vi "Terminals - Filter Left-Top Term.vi"(11 "Terms[]":refnum<vi>[](array[refnum])) -> (3 "Terms[] out":refnum<vi>[](array[refnum]))   [LabVIEW 2020, in "CSM-Helper.lvclass"]
uses:
  CSM-Helper.lvclass
  CSM-Helper.lvclass/CSM-Helper.ctl
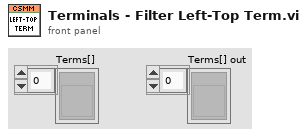
[diagram p1: front panel]
types:
  T1 = typedef "LVPositionTypeDef.ctl" = cluster{"Left":i32, "Top":i32}
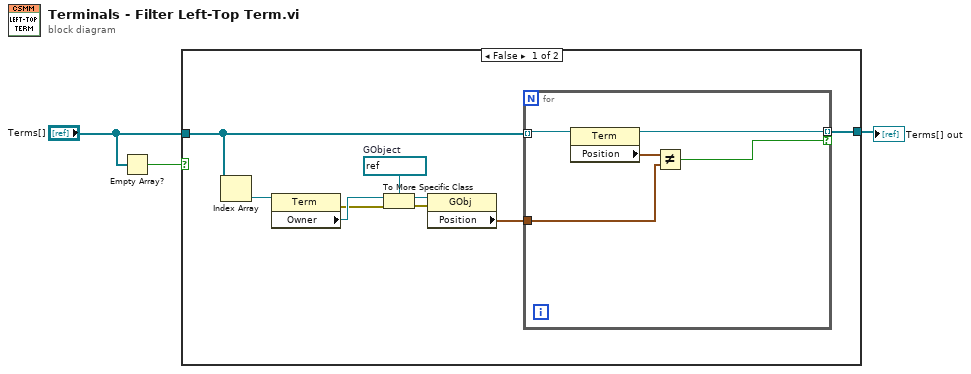
[diagram p0: block diagram]
diagram:
  n1 = Empty Array?(array="Terms[]") -> (empty?=w2:bool)
  n2 = case shown="False" w2 {
    tunnel: "Terms[]" -> [w12 w18]
    tunnel: [w11 w18] -> w1
    frame False {
      w4 = refnum<vi> refnum  # GObject
      n3 = Index Array(array=w12) -> (element=w9:refnum<vi>)  [unwired: 1 in]
      n4 = property class="Term"(reference=w9) -> (error out=w5:errorcluster, "Owner"=w8:refnum<vi>)  [unwired: 1 in, 1 out]
      n5 = To More Specific Class(target class=w4, reference=w8, error in=w5) -> (specific class reference=w7:refnum<vi>, error out=w6:errorcluster)
      n6 = property class="GObj"(reference=w7, error in=w6) -> ("Position"=w10:T1)  [unwired: 2 out]
      n7 = for {
        tunnel: w12 -> [w17] mode=indexing
        tunnel: [w16] -> w11 mode=indexing if=w13
        tunnel: w10 -> [w14]
        n8 = property class="Term"(reference=w17) -> (reference out=w16:refnum<vi>, "Position"=w15:T1)  [unwired: 1 in, 1 out]
        n9 = Not Equal?(x=w15, y=w14) -> (x != y?=w13:bool)
      }
    }
    frame True {
    }
  }
  "Terms[] out" <- w1
